vi "FGV_OEE_SQL_raw_data.vi"(7 "options":T2=enum."get_all_info", 8 "error_in":errorcluster, 11 "input":variant) -> (0 "error_out":errorcluster, 3 "SQL_raw_data_out":T1)   [LabVIEW 2019]
uses:
  FGV_OEE_SQL_raw_data.ctl
  OEE_SQL_raw_data.ctl
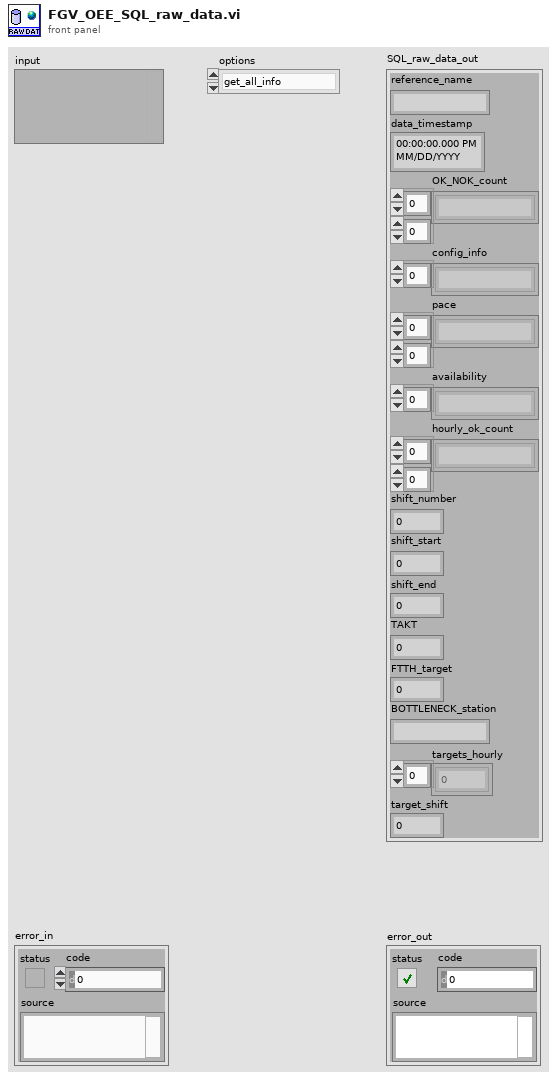
[diagram p1: front panel]
types:
  T1 = typedef "OEE_SQL_raw_data.ctl" = cluster{"reference_name":string, "data_timestamp":timestamp, "OK_NOK_count":string[][], "config_info":string[], "pace":string[][], "availability":string[], "hourly_ok_count":string[][], "shift_number":i8, "shift_start":i8, "shift_end":i8, "TAKT":u16, "FTTH_target":u16, "BOTTLENECK_station":string, "targets_hourly":u16[], "target_shift":u16}
  T2 = typedef "FGV_OEE_SQL_raw_data.ctl" = enum16{"initialize", "set_reference_name", "set_timestamp", "set_OK_NOK_count", "set_config_info", "set_pace", "set_availability", "set_hourly_ok_count", "set_targets", "get_all_info"}
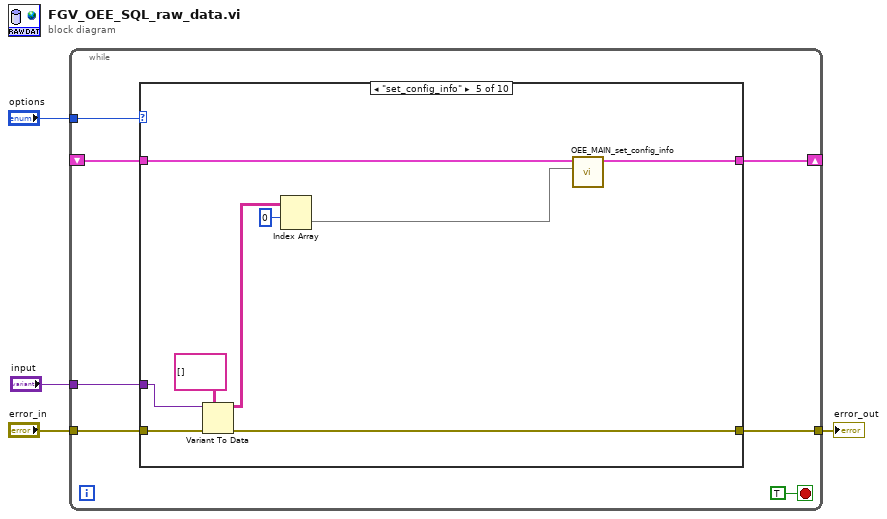
[diagram p0: block diagram]
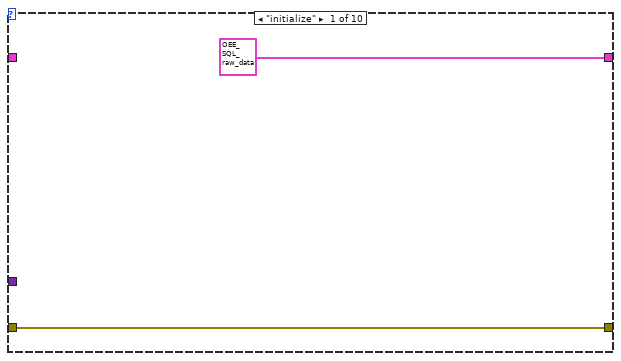
[diagram p2: hidden frame]
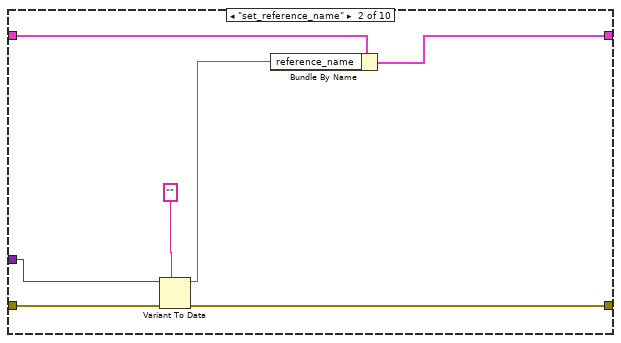
[diagram p3: hidden frame]
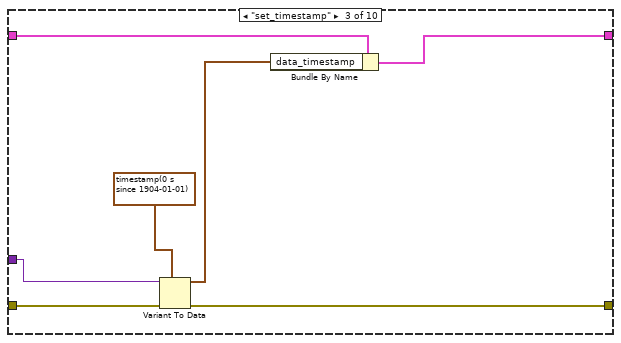
[diagram p4: hidden frame]
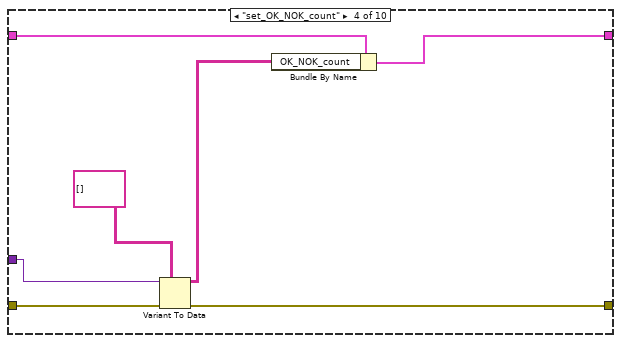
[diagram p5: hidden frame]
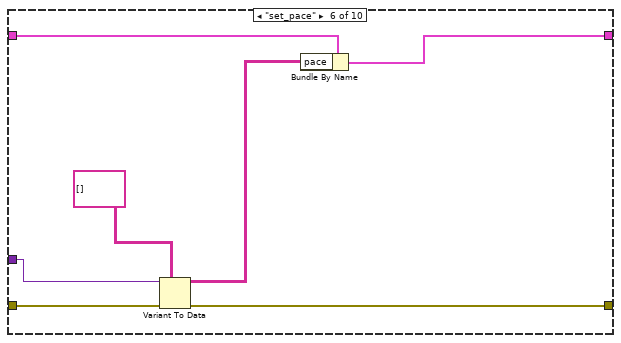
[diagram p6: hidden frame]
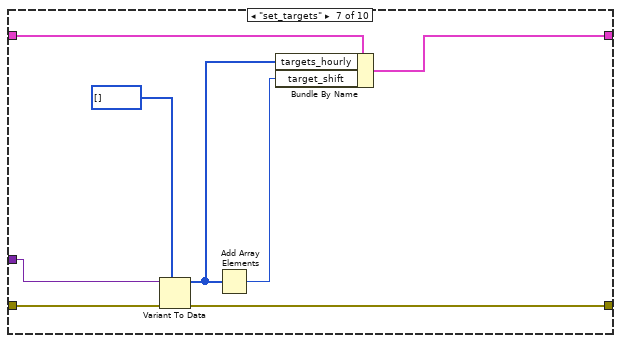
[diagram p7: hidden frame]
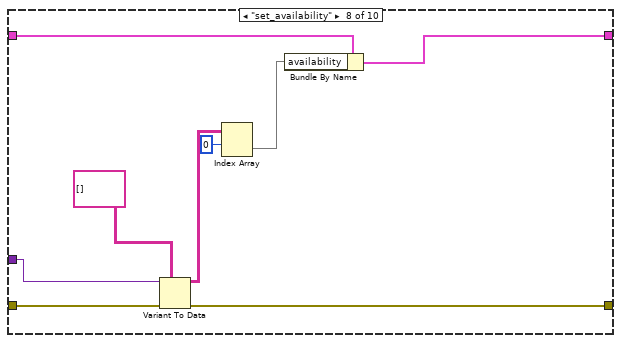
[diagram p8: hidden frame]
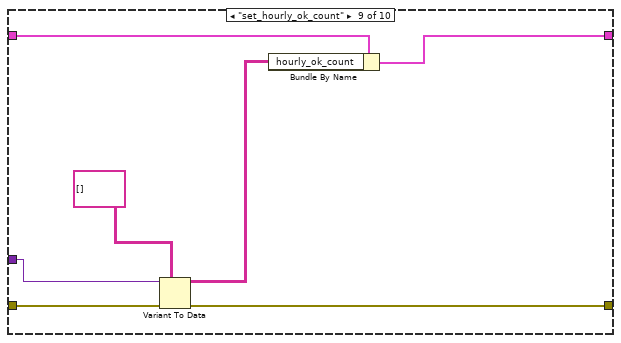
[diagram p9: hidden frame]
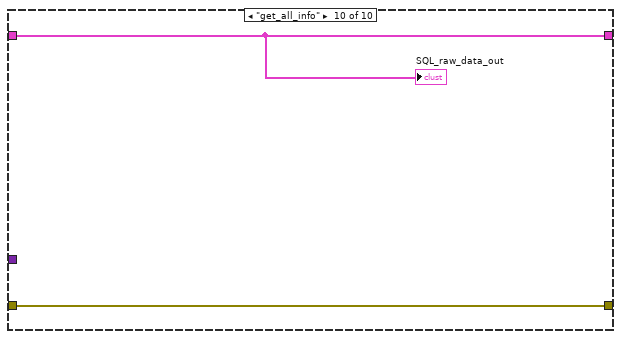
[diagram p10: hidden frame]
diagram:
  n1 = while {
    tunnel: "options" -> [w10]
    tunnel: [w9] -> w3
    tunnel: "error_in" -> [w8]
    shift-right: [w7] -> _
    shift-left: _ -> [w6]
    tunnel: "input" -> [w5]
    stop <- TRUE stop-if-true
    n2 = case shown="\"set_config_info\"" w10 {
      tunnel: [w13 w19 w26 w32 w41 w48 w57 w65 w72 w76] -> w9
      tunnel: w8 -> [w13 w20 w27 w33 w42 w49 w58 w66 w73 w76]
      tunnel: [T1 {"reference_name"="", "data_timestamp"=timestamp(0 s since 1904-01-01), "OK_NOK_count"=[], "config_info"=[], "pace"=[], "availability"=[], "hourly_ok_count"=[], "shift_number"=0, "shift_start"=0, "shift_end"=0, "TAKT"=0, "FTTH_target"=0, "BOTTLENECK_station"="", "targets_hourly"=[], "target_shift"=0} ("SQL_raw_data_in") w16 w24 w29 w39 w46 w55 w63 w70 w75] -> w7
      tunnel: w6 -> [_ w18 w25 w31 w40 w47 w56 w64 w71 w75]
      tunnel: w5 -> [_ w15 w23 w28 w38 w45 w54 w62 w69 _]
      frame "initialize" {
      }
      frame "set_reference_name" {
        n3 = Variant To Data(error in=w20, type="", Variant=w15) -> (data=w17:string, error out=w19:errorcluster)
        n4 = Bundle By Name(cluster=w18, "reference_name"=w17) -> (w16:T1)
      }
      frame "set_timestamp" {
        n5 = Variant To Data(error in=w27, type=timestamp(0 s since 1904-01-01) ("current time"), Variant=w23) -> (data=w21:timestamp, error out=w26:errorcluster)
        n6 = Bundle By Name(cluster=w25, "data_timestamp"=w21) -> (w24:T1)
      }
      frame "set_OK_NOK_count" {
        n7 = Variant To Data(error in=w33, type=string[][] [], Variant=w28) -> (data=w30:string[][], error out=w32:errorcluster)
        n8 = Bundle By Name(cluster=w31, "OK_NOK_count"=w30) -> (w29:T1)
      }
      frame "set_config_info" {
        n9 = Variant To Data(error in=w42, type=string[][] [], Variant=w38) -> (data=w37:string[][], error out=w41:errorcluster)
        n10 = Index Array(array=w37, index (row)=0) -> (element=w35:string[])  [unwired: 1 in]
        n11 = call "OEE_MAIN_set_config_info.vi"("Array"=w35, "SQL_raw_data_in"=w40) -> ("SQL_raw_data_out"=w39:T1)  [unwired: 9 in]
      }
      frame "set_pace" {
        n12 = Variant To Data(error in=w49, type=string[][] [], Variant=w45) -> (data=w44:string[][], error out=w48:errorcluster)
        n13 = Bundle By Name(cluster=w47, "pace"=w44) -> (w46:T1)
      }
      frame "set_targets" {
        n14 = Variant To Data(error in=w58, type=u16[] [] ("unsigned 16bit integer"), Variant=w54) -> (data=w52:u16[], error out=w57:errorcluster)
        n15 = Add Array Elements(numeric array=w52) -> (sum=w51:u16)
        n16 = Bundle By Name(cluster=w56, "targets_hourly"=w52, "target_shift"=w51) -> (w55:T1)
      }
      frame "set_availability" {
        n17 = Variant To Data(error in=w66, type=string[][] [], Variant=w62) -> (data=w61:string[][], error out=w65:errorcluster)
        n18 = Index Array(array=w61, index (row)=0) -> (element=w59:string[])  [unwired: 1 in]
        n19 = Bundle By Name(cluster=w64, "availability"=w59) -> (w63:T1)
      }
      frame "set_hourly_ok_count" {
        n20 = Variant To Data(error in=w73, type=string[][] [], Variant=w69) -> (data=w68:string[][], error out=w72:errorcluster)
        n21 = Bundle By Name(cluster=w71, "hourly_ok_count"=w68) -> (w70:T1)
      }
      frame "get_all_info" {
        "SQL_raw_data_out" <- w75
      }
    }
  }
  "error_out" <- w3
